vi "Launch Event Handlers.vi"(8 "error in (no error)":errorcluster, 11 "IViewable In":refnum<class "IViewable.lvclass">) -> (0 "error out":errorcluster, 3 "IViewable Out":refnum<class "IViewable.lvclass">)   [LabVIEW 2017, in "IViewable.lvlib" / "IViewable.lvclass"]
uses:
  <vilib>/gpm_packages/@cs/mva-viewable/Source/IViewable/IViewable/IViewable.lvclass
  <vilib>/gpm_packages/@cs/mva-viewable/Source/ActorEvents/IEventAggregator/IEventAggregator.lvclass
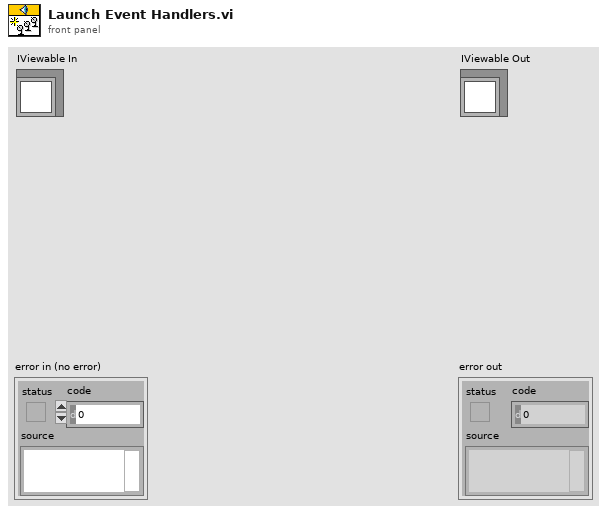
[diagram p1: front panel]
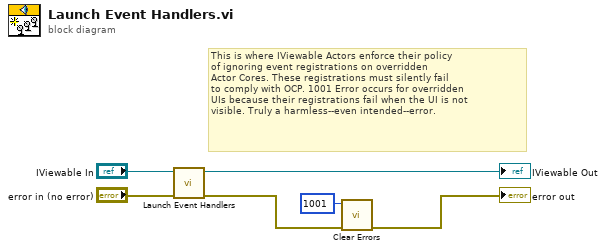
[diagram p0: block diagram]
diagram:
  # "This is where IViewable Actors enforce their policy\nof ignoring event registrations on overridden\nActor Cores. These registrations must silently fail\nto comply with OCP. 1001 Error occurs for overridden\nUIs because their registrations fail when the UI is not\nvisible. Truly a harmless--even intended--error."
  n1 = call-parent "Launch Event Handlers.vi"("error in (no error)"="error in (no error)", "IEventAggregator In"="IViewable In") -> ("error out"=w4:errorcluster, "IEventAggregator Out"=→"IViewable Out":refnum<class "IViewable.lvclass">)  [unwired: 8 in]
  n2 = call <vilib>:"Clear Errors.vi"("error in (no error)"=w4, "specific error code to clear (0: all)"=1001) -> ("error out"=→"error out":errorcluster)  [unwired: 4 in, 1 out]
